vi "Toptica-Parse_param-disp.vi"() -> ()   [LabVIEW 2011]
panel:
  out "Array":cluster{string, "String 1":string}[](array[cluster])
  out "String Array":string[](array[string])
  in  "param-disp":string="laser1\n  :label = \"640 nm\"\n  :type = \"640nm laser diode\"\n  :enable = #f\n  :cw = #f\n  :ready = #t\n  :fault = #f\n  :clip = #f\n  :status = 4097\n  :status-txt = \"AVAILABLE USETTL\"\n  :level = 100\n  :analog-mode = #f\n  :use-ttl = #t\n  :fine\n    :enable = #t\n    :a = 70.5882\n    :b = 30.1961\n  :delay = 170\n  :entime = 1215120\n  :entime-txt = \"337:32:00\"\n  :ontime = 120781\n  :ontime-txt = \"33:33:01\"\n  :beam\nlaser2\n  :label = \"561 nm\"\n  :type = \"FDDL_561\"\n  :enable = #t\n  :cw = #f\n  :ready = #t\n  :fault = #f\n  :clip = #f\n  :status = 4099\n  :status-txt = \"AVAILABLE ENABLED USETTL\"\n  :level = 100\n  :analog-mode = #f\n  :use-ttl = #t\n  :fine\n    :enable = #t\n    :a = 36.8627\n    :b = 3.52941\n  :delay = 170\n  :entime = 782372\n  :entime-txt = \"217:19:32\"\n  :ontime = 178489\n  :ontime-txt = \"49:34:49\"\n  :shg\n    :temp = 29.102 -> 29.1\n  :beam\nlaser3\n  :label = \"488 nm\"\n  :type = \"488nm laser diode\"\n  :enable = #t\n  :cw = #f\n  :ready = #t\n  :fault = #f\n  :clip = #f\n  :status = 4099\n  :status-txt = \"AVAILABLE ENABLED USETTL\"\n  :level = 100\n  :analog-mode = #f\n  :use-ttl = #t\n  :fine\n    :enable = #t\n    :a = 70.1961\n    :b = 10.1961\n  :delay = 170\n  :entime = 1247813\n  :entime-txt = \"346:36:53\"\n  :ontime = 211459\n  :ontime-txt = \"58:44:19\"\n  :beam\nlaser4\n  :label = \"405 nm\"\n  :type = \"405nm laser diode\"\n  :enable = #t\n  :cw = #f\n  :ready = #t\n  :fault = #f\n  :clip = #f\n  :status = 4099\n  :status-txt = \"AVAILABLE ENABLED USETTL\"\n  :level = 99.8779\n  :analog-mode = #f\n  :use-ttl = #t\n  :fine\n    :enable = #t\n    :a = 70.1961\n    :b = 10.1961\n  :delay = 170\n  :entime = 1443557\n  :entime-txt = \"400:59:17\"\n  :ontime = 135946\n  :ontime-txt = \"37:45:46\"\n  :beam\nall\n  :enable = #f\n  :enable-led = #t\n  :cw = #f\n  :analog-mode = #f\n  :use-ttl = #t\n  :ttl-active-high = #t\n  :ttl-master-mode = #f\n  :digital-over-analog = #t\n  :ready = #t\n  :fault = #f\ntec-d\n  :enable = #t\n  :status = 7\n  :status-txt = \"ENABLED TEMPOK HEATING\"\n  :fault = #f\n  :temp = 31.949 -> 32\ntec-l\n  :enable = #t\n  :status = 7\n  :status-txt = \"ENABLED TEMPOK HEATING\"\n  :fault = #f\n  :temp = 25.031 -> 25\ndx5100\n  :serial-number = \"#S406 14.04.2014\"\n  :fw-ver = \"07/20/15 10:21:36 DX5100.346\"\ntec-c\n  :enable = #t\n  :status = 7\n  :status-txt = \"ENABLED TEMPOK HEATING\"\n  :temp = 29.1013 -> 29.1\n  :current = 0\n  :voltage = 0.000143536\n  :temp-min = 18\n  :temp-max = 55\n  :kp = 0.3\n  :ki = 0.1\n  :kd = 0\n  :calibration = (#f 0.00110459 0.00023545 1.03481e-07 0 0 0)\ntec-p\n  :enable = #t\n  :status = 11\n  :status-txt = \"ENABLED TEMPOK COOLING\"\n  :temp = 18.0015 -> 18\n  :current = 0.169922\n  :voltage = 0.000159429\n  :temp-min = 15\n  :temp-max = 35\n  :kp = 0.3\n  :ki = 0.1\n  :kd = 0\n  :calibration = (#f 0.00110459 0.00023545 1.03481e-07 0 0 0)\npowermon\n  :cal = 0\n  :cal-udelay = 0\n  :signal = 21\n  :signal-source = \"int\"\ninterlock = #f\nbase-temp = 'Error -16'\nbuzzer\n  :welcome = \" \"\ntan = 0\nuptime = 2269207\nuptime-txt = \"630:20:07\"\ntime = \"2017-03-20 16:34:29\"\nfw-ver = \"1.0.0.7\"\ndecof-ver = \"3.1.1476\"\nserial-number = \"iCHROME_CLE_TILL_Prototyp1\"\nsystem-type = \"MLE-Young\"\nsystem-model = \"DDDD\"\nsystem-label = \"\"\nul = 3\nnet-conf\n  :ip-addr = \"192.168.2.2\"\n  :net-mask = \"255.255.255.0\"\n  :mac-addr = \"00:0C:C6:7F:02:4B\"\n  :dhcp = #f\n  :cmd-port = 50000\n  :mon-port = 0\necho = #t\nscript\n  :boot\n    :busy = #f\n    :size = 52\n  :console\n    :busy = #f\n    :size = 0\n  :misc\n    :busy = #f\n    :size = 5532"
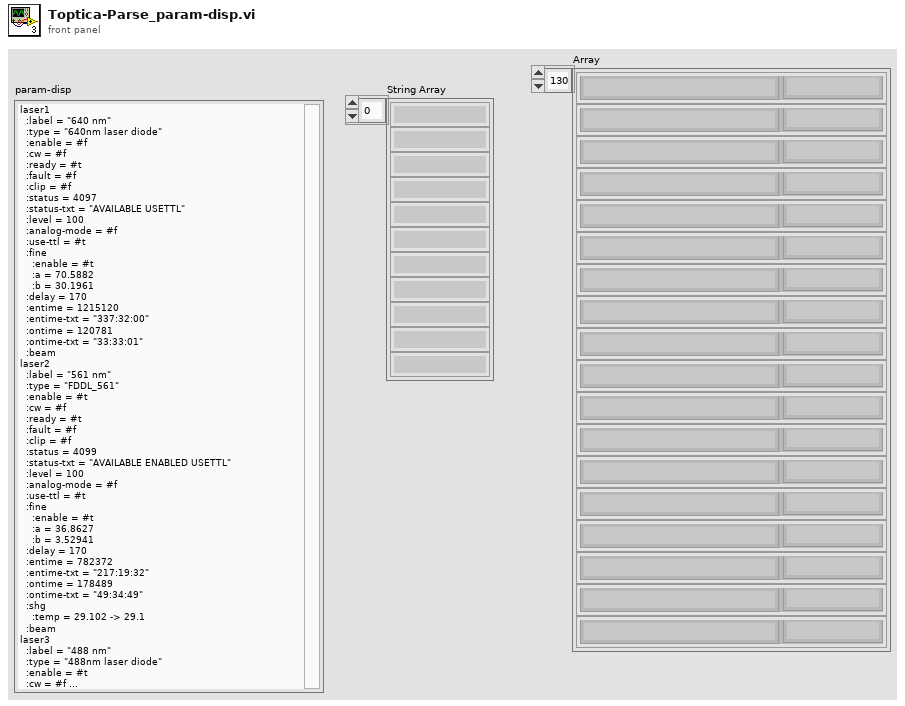
[diagram p1: front panel]
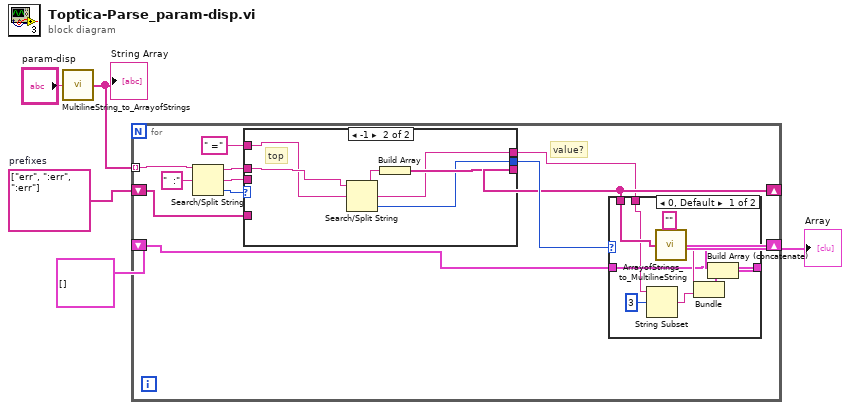
[diagram p0: block diagram]
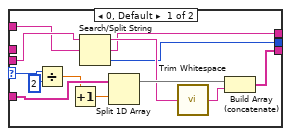
[diagram p3: hidden frame]
diagram:
  w1 = string[] ["err", ":err", ":err"]  # prefixes
  n1 = call "MultilineString_to_ArrayofStrings.vi"("String 1"="param-disp") -> ("String Array"=w4:string[])  [unwired: 1 in]
  "String Array" <- w4
  n2 = for {
    tunnel: w4 -> [w16] mode=indexing
    shift-right: [w8] -> _
    shift-left: w1 -> [w12]
    shift-right: [w9] -> w2
    shift-left: cluster{string, "String 1":string}[] [] -> [w10]
    # "value?"
    n3 = Search/Split String(string=w16, search string/char (-)="  :") -> (substring before match=w14:string, match + rest of string=w13:string, offset of match=w15:i32)  [unwired: 1 in]
    n4 = case shown="-1" w15 {
      selector: w15 -> [w40 _]
      tunnel: w14 -> [_ w45]
      tunnel: w13 -> [w38 _]
      tunnel: [w32 w46] -> w8
      tunnel: w12 -> [w37 _]
      tunnel: [w31 w44] -> w7
      tunnel: [w30 w43] -> w11
      tunnel: " =" ("regular expression") -> [w28 w42]
      frame 0, Default {
        n5 = Divide(x=w40, y=2) -> (x/y=w36:dbl)
        n6 = Increment(x=w36) -> (x+1=w35:dbl)
        n7 = Search/Split String(string=w38, search string/char (-)=w28) -> (substring before match=w33:string, match + rest of string=w31:string, offset of match=w30:i32)  [unwired: 1 in]
        n8 = Split 1D Array(array=w37, index=w35) -> (first subarray=w34:string[])  [unwired: 1 out]
        n9 = call <vilib>:"Trim Whitespace.vi"("string"=w33) -> ("trimmed string"=w29:string)  [unwired: 1 in]
        n10 = Build Array (concatenate)(w34, w29) -> (w32:string[])
      }
      frame -1 {
        # "top"
        n11 = Search/Split String(string=w45, search string/char (-)=w42) -> (substring before match=w41:string, match + rest of string=w44:string, offset of match=w43:i32)  [unwired: 1 in]
        n12 = Build Array(w41) -> (w46:string[])
      }
    }
    n13 = case shown="0, Default" w11 {
      tunnel: w10 -> [w23 w27]
      tunnel: [w21 w27] -> w9
      tunnel: w8 -> [w26 _]
      tunnel: w7 -> [w20 _]
      frame 0, Default {
        n14 = String Subset(string=w20, offset (0)=3) -> (substring=w19:string)  [unwired: 1 in]
        n15 = call "ArrayofStrings_to_MultilineString.vi"("String Array"=w26, "NewLineString"="") -> ("String 1"=w24:string)
        n16 = Bundle("String 1"=w24, "String 1"=w19) -> (w22:cluster{"String 1":string, "String 1":string})  [unwired: 1 in]
        n17 = Build Array (concatenate)(w23, w22) -> (w21:cluster{"String 1":string, "String 1":string}[])
      }
      frame -1 {
      }
    }
  }
  "Array" <- w2
